vi "Set Message Class Icon.vi"(8 "error in (no error)":errorcluster, 9 "Icon in":refnum<class "Icon.lvclass">, 10 "New Class Path":path, 11 "AppInst":refnum<vi>) -> (0 "error out":errorcluster, 1 "Icon out":refnum<class "Icon.lvclass">)   [LabVIEW 2020, in "Message Maker.lvlib"]
uses:
  Message Maker.lvlib
  <vilib>/LabVIEW Icon API/LabVIEW Icon API.lvlib
  <vilib>/LabVIEW Icon API/lv_icon/Classes/Icon/Icon.lvclass
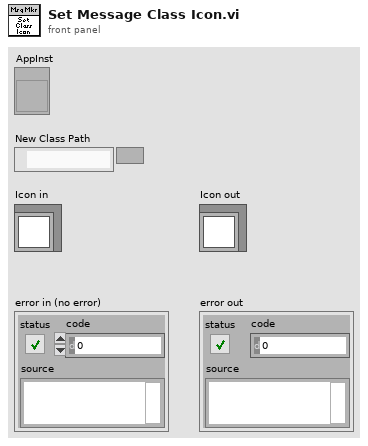
[diagram p1: front panel]
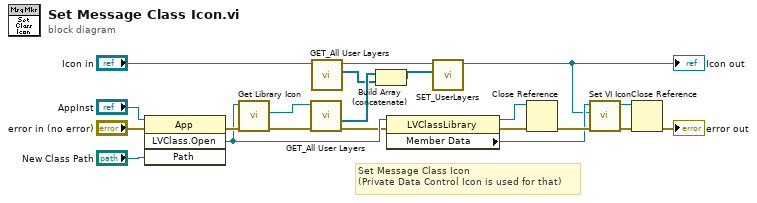
[diagram p0: block diagram]
diagram:
  # "Set Message Class Icon\n(Private Data Control Icon is used for that)"
  n1 = invoke class="App" method="LVClass.Open"(reference="AppInst", error in="error in (no error)", "Path"="New Class Path") -> (error out=w12:errorcluster, "LVClass.Open"=w9:refnum<vi>)  [unwired: 1 in, 2 out]
  n2 = call <vilib>:"Get Library Icon.vi"("error in (no error)"=w12, "Library Refnum in"=w9) -> ("error out"=w7:errorcluster, "Icon"=w8:refnum<class "Icon.lvclass">)  [unwired: 7 in, 1 out]
  n3 = call-dynamic "GET_All User Layers.vi"("error in (no error)"=w7, "Icon.lvclass in"=w8) -> ("error out"=w6:errorcluster, "User Layer"=w5:refnum<class "Layer.lvclass">[])  [unwired: 7 in, 1 out]
  n4 = call-dynamic "GET_All User Layers.vi"("Icon.lvclass in"="Icon in") -> ("User Layer"=w1:refnum<class "Layer.lvclass">[], "Icon.lvclass out"=w3:refnum<class "Icon.lvclass">)  [unwired: 8 in, 1 out]
  n5 = Build Array (concatenate)(w5, w1) -> (w2:refnum<class "Layer.lvclass">[])
  n6 = property class="LVClassLibrary"(reference=w9, error in=w6) -> (reference out=w15:refnum<vi>, error out=w14:errorcluster, "Member Data"=w16:refnum<vi>)
  n7 = call-dynamic "SET_UserLayers.vi"("Layers"=w2, "Icon.lvclass in"=w3) -> ("Icon.lvclass out"=w4:refnum<class "Icon.lvclass">)  [unwired: 8 in, 1 out]
  "Icon out" <- w4
  n8 = Close Reference(reference=w15, error in (no error)=w14) -> (error out=w17:errorcluster)
  n9 = call <vilib>:"Set VI Icon.vi"("error in (no error)"=w17, "Icon"=w4, "VI Refnum in"=w16) -> ("error out"=w19:errorcluster, "VI Refnum out"=w18:refnum<vi>)  [unwired: 7 in]
  n10 = Close Reference(reference=w18, error in (no error)=w19) -> (error out=→"error out":errorcluster)
